vi "XmlRpc.vi"() -> ()   [LabVIEW 2022 SP3]
uses:
  C:/Users/fg/Documents/UniversalRobots.vi/LabVIEW_2024/UnderAutomation.UniversalRobots/lib/UnderAutomation.UniversalRobots.dll
  LabVIEW_2024/UnderAutomation.UniversalRobots/lib/UnderAutomation.UniversalRobots.dll
panel:
  in  "stop":bool
  in  "Answer number":dbl
  # "XML-RPC server sample"
  # "Here is an example of code to run in the robot :\n\nrpc:=rpc_factory(\"xmlrpc\",\"http://IP_OF_THIS_MACHINE:50000\")\nanswerPose:=rpc.GetPose()\nanswerOther:=rpc.get_answer(\"Hello\", True, False, 12, 12.2, p[100,100,120,0.1,0,0], [12,1.2,123])"
  # "If method is GetPose(), answer p[0.1, -0.2, 0.2]\n\nFor all other methods, answer this number :"
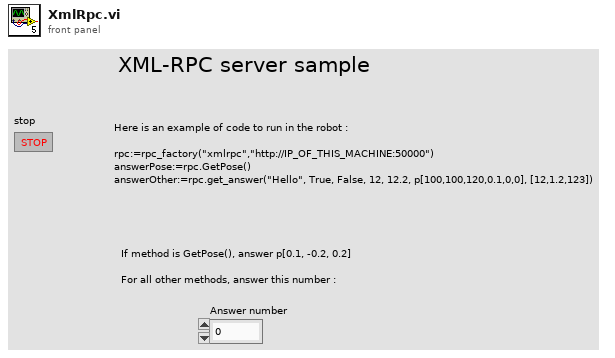
[diagram p1: front panel]
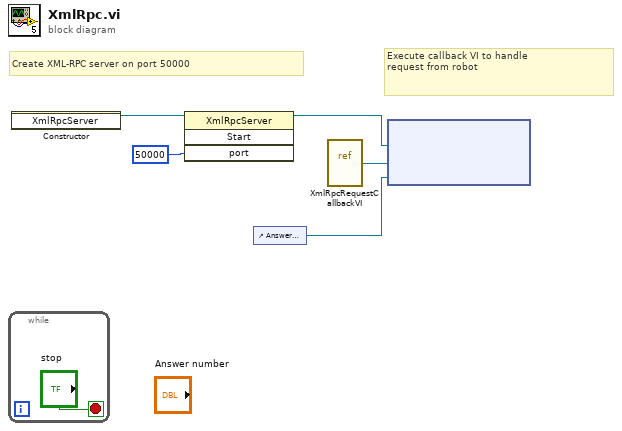
[diagram p0: block diagram]
diagram:
  # "Execute callback VI to handle\nrequest from robot"
  # "Create XML-RPC server on port 50000"
  n1 = while {
    stop <- "stop" stop-if-true
  }
  n2 = constructor class="XmlRpcServer"() -> (reference out=w5:refnum<k24>)  [unwired: 3 in, 2 out]
  n3 = invoke class="XmlRpcServer" method="Start"(reference=w5, "port"=50000) -> (reference out=w3:refnum<k24>)  [unwired: 2 in, 3 out]
  n4 = control-ref of="Answer number"() -> (w2:refnum<vi>)
  n5 = vi-ref "XmlRpcRequestCallbackVI.vi"() -> ("vi reference"=w1:refnum<vi>)
  n6 = node(w3, w1, w2) -> ()  [unwired: 2 in, 2 out]
